vi "DelTaskbarIcon.vi"(4 "error in (no error)":errorcluster, 6 "uID (1)":i32=1, 7 "hWnd (NULL)":T1) -> (0 "error out":errorcluster)   [LabVIEW 2011]
uses:
  WinUSER/Windows/hWnd.ctl
  NOTIFYICONDATA.ctl
  NOTIFYICON_OPERATIONS.ctl
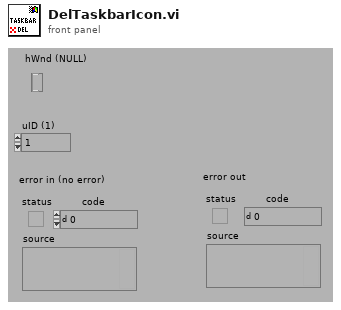
[diagram p1: front panel]
types:
  T1 = typedef "hWnd.ctl" = refnum<k1>
  T2 = typedef "NOTIFYICON_OPERATIONS.ctl" = enum16{"NIM_ADD", "NIM_MODIFY", "NIM_DELETE", "NIM_SETFOCUS", "NIM_SETVERSION"}
  T3 = typedef "NOTIFYICONDATA.ctl" = cluster{"cbSize":i32, "hWnd":i32, "uID":i32, "uFlags":i32, "uCallbackMessage":i32, "hIcon":i32, "szTip[64]":string}
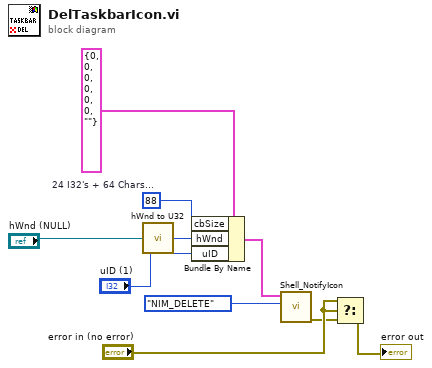
[diagram p0: block diagram]
diagram:
  w9 = 88  # 24 I32's + 64 Chars...
  n1 = call "hWnd to U32.vi"("hWnd"="hWnd (NULL)") -> ("hWnd"=w4:u32)  [unwired: 4 out]
  n2 = Bundle By Name(cluster=T3 {"cbSize"=0, "hWnd"=0, "uID"=0, "uFlags"=0, "uCallbackMessage"=0, "hIcon"=0, "szTip[64]"=""} ("NOTIFYICONDATA"), "cbSize"=w9, "hWnd"=w4, "uID"="uID (1)") -> (w8:T3)
  n3 = call "Shell_NotifyIcon.vi"("Operation (NIF_ADD)"=NOTIFYICON_OPERATIONS."NIM_DELETE", "NOTIFYICONDATA"=w8) -> ("error out"=w2:errorcluster)  [unwired: 1 in, 4 out]
  n4 = Select(t="error in (no error)", s="error in (no error)", f=w2) -> (s? t:f=→"error out":errorcluster)
